vi "Finish timed acq.vi"(8 "error in (no error)":errorcluster, 11 "Queue in":refnum<queue>) -> (0 "error out":errorcluster)   [LabVIEW 2020]
uses:
  Message Queue/Message Queue.lvlib
  Message Queue/Enqueue Message (Single).vi
  Message Queue/Message Cluster.ctl
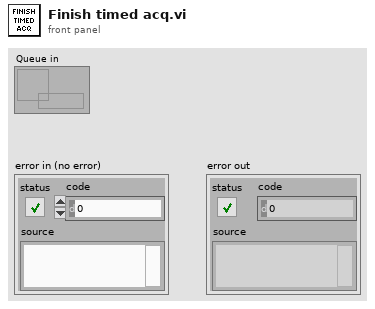
[diagram p1: front panel]
types:
  T1 = enum8{"Enabled", "Disabled", "Disabled and Grayed Out"}[]
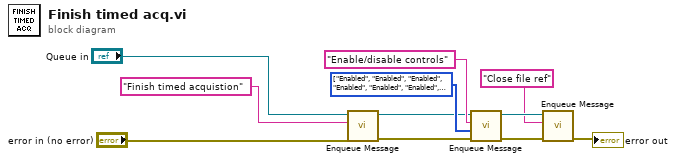
[diagram p0: block diagram]
diagram:
  w7 = T1 [enum."Enabled", enum."Enabled", enum."Enabled", enum."Enabled", enum."Enabled", enum."Enabled", enum."Enabled", enum."Enabled", enum."Disabled and Grayed Out", enum."Enabled", enum."Enabled", enum."Enabled"] items=["Enabled", "Disabled", "Disabled and Grayed Out"] ("Disabled")
  n1 = call-poly "Enqueue Message.vi"("error in (no error)"="error in (no error)", "Message"="Finish timed acquistion", "Message Queue"="Queue in") -> ("error out"=w4:errorcluster, "dup Message Queue"=w5:refnum<queue>)  [unwired: 7 in]
  n2 = call-poly "Enqueue Message.vi"("error in (no error)"=w4, "Message Data"=w7, "Message"="Enable/disable controls", "Message Queue"=w5) -> ("error out"=w8:errorcluster, "dup Message Queue"=w11:refnum<queue>)  [unwired: 6 in]
  n3 = call-poly "Enqueue Message.vi"("error in (no error)"=w8, "Message"="Close file ref", "Message Queue"=w11) -> ("error out"=→"error out":errorcluster)  [unwired: 7 in, 1 out]
